vi "Write Sample Rate.vi"(8 "error in (no error)":errorcluster, 10 "sample rate [Hz]":dbl=51200.0, 11 "signal configuration":refnum<class "SV Signal.lvclass">) -> (0 "error out":errorcluster, 3 "signal configuration":refnum<class "SV Signal.lvclass">)   [LabVIEW 2017, in "SV Signal.lvclass"]
uses:
  <vilib>/addons/_NISVFA/_Generation/Signal Generation/SV Signal/SV Signal.lvclass
  <vilib>/addons/_NISVFA/_Generation/Signal Generation/SV Signal/SV Signal.lvclass/SV Signal.ctl
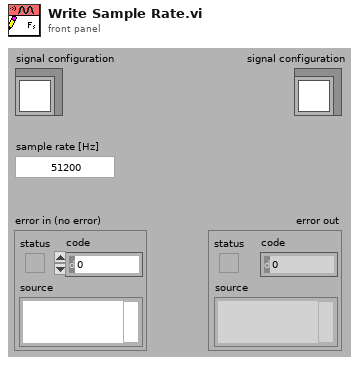
[diagram p1: front panel]
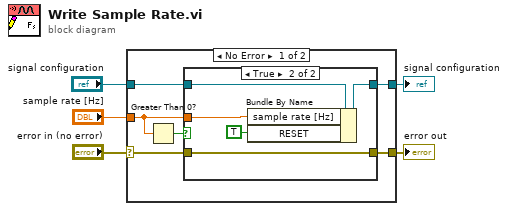
[diagram p0: block diagram]
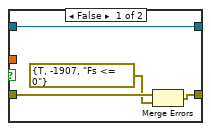
[diagram p2: hidden frame]
diagram:
  n1 = case shown="No Error" "error in (no error)" {
    selector: "error in (no error)" -> [w7 w21]
    tunnel: [w6 w21] -> w4
    tunnel: [w10 w22] -> w2
    tunnel: "signal configuration" -> [w11 w22]
    tunnel: "sample rate [Hz]" -> [w9 _]
    frame No Error {
      n2 = Greater Than 0?(x=w9) -> (x > 0?=w8:bool)
      n3 = case shown="True" w8 {
        tunnel: w11 -> [w15 w20]
        tunnel: [w15 w19] -> w10
        tunnel: w9 -> [_ w18]
        tunnel: w7 -> [w14 w17]
        tunnel: [w12 w17] -> w6
        frame False {
          n4 = Merge Errors(w14, errorcluster {"status"=TRUE, "code"=-1907, "source"="Fs <= 0"} ("error in (no error)")) -> (w12:errorcluster)
        }
        frame True {
          n5 = Bundle By Name(cluster=w20, "sample rate [Hz]"=w18, "RESET"=TRUE ("state.RESET")) -> (w19:refnum<class "SV Signal.lvclass">)
        }
      }
    }
    frame Error {
    }
  }
  "error out" <- w4
  "signal configuration" <- w2
